vi "WPI_AccumulatorGetOutput.vi"(8 "error in (no error)":errorcluster, 11 "AIDeviceRef":T1={"DevStatus"={"status"=FALSE, "code"=0, "source"=""}, "Analog Channel"=enum."Invalid"}) -> (0 "error out":errorcluster, 1 "Duration (Seconds)":dbl, 2 "Value (Volt Seconds)":dbl, 3 "AIDeviceRef":T1={"DevStatus"={"status"=FALSE, "code"=0, "source"=""}, "Analog Channel"=enum."Invalid"})   [LabVIEW 2017]
doc: "Returns the current value of the accumulator on the FPGA on the robotRIO device. The GetOutput VI also returns the number of seconds that has passed since the accumulator was last reset. You can use this VI to perform averaging.\n\nThis software is licensed. Open the labview\\readme\\WPI Robotics Library Open Source License.txt file for more information."
uses:
  <vilib>/Rock Robotics/WPI/AnalogChannel/WPI_AnalogChannelDevRef.ctl
  <vilib>/Rock Robotics/SystemInterfaces/AI/FPGA_AIChannel.ctl
  <vilib>/Rock Robotics/SystemInterfaces/System/FPGA_SystemGet.vi
  <vilib>/Rock Robotics/SystemInterfaces/AI/FPGA_AIAverageBits.vi
  <vilib>/Rock Robotics/SystemInterfaces/AI/FPGA_AIERRInvalidAnalogChannel.vi
  <vilib>/Rock Robotics/SystemInterfaces/AI/FPGA_AIOversampleBits.vi
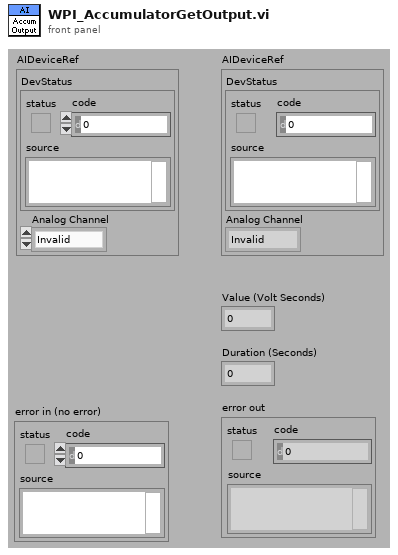
[diagram p1: front panel]
types:
  T1 = typedef "WPI_AnalogChannelDevRef.ctl" = cluster{"DevStatus":errorcluster, "Analog Channel":T2}
  T2 = typedef "FPGA_AIChannel.ctl" = enum8{"AI 0", "AI 1", "AI 2", "AI 3", "AI MXP 0", "AI MXP 1", "AI MXP 2", "AI MXP 3", "Invalid"}
  T3 = typedef "FPGA_AIDevRef.ctl" = cluster{"DevStatus":errorcluster}
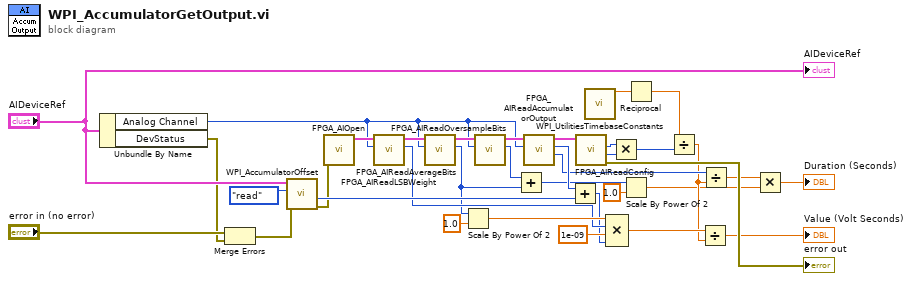
[diagram p0: block diagram]
diagram:
  n1 = Unbundle By Name("AIDeviceRef") -> ("Analog Channel"=w14:T2, "DevStatus"=w2:errorcluster)
  n2 = Merge Errors("error in (no error)", w2) -> (w1:errorcluster)
  n3 = call <vilib>:"WPI_AccumulatorOffset.vi"("error in (no error)"=w1, "Action"=enum16{"read", "write"}."read" ("what do"), "AIDeviceRef"="AIDeviceRef") -> ("error out"=w6:errorcluster, "Offset Out"=w31:i32)  [unwired: 1 in, 6 out]
  n4 = call <vilib>:"FPGA_AIOpen.vi"("error in (no error)"=w6) -> ("AI Reference out"=w28:T3)  [unwired: 2 in, 8 out]
  n5 = call <vilib>:"FPGA_AIReadLSBWeight.vi"("Channel"=w14, "AI Reference"=w28) -> ("LSBWeight"=w24:u32, "AI Reference"=w29:T3)  [unwired: 1 in, 7 out]
  n6 = call <vilib>:"FPGA_AIReadAverageBits.vi"("Channel"=w14, "AI Reference in"=w29) -> ("AverageBits"=w12:u8, "AI Reference out"=w16:T3)  [unwired: 1 in, 7 out]
  n7 = Scale By Power Of 2(n=w12, x=1.0) -> (x*2^n=w26:dbl)
  n8 = call <vilib>:"FPGA_AIReadOversampleBits.vi"("Channel"=w14, "AI Reference in"=w16) -> ("OversampleBits"=w13:u8, "AI Reference out"=w15:T3)  [unwired: 2 in, 6 out]
  n9 = Add(x=w13, y=w12) -> (x+y=w10:u8)
  n10 = call <vilib>:"FPGA_AIReadAccumulatorOutput.vi"("Channel"=w14, "AI Reference"=w15) -> ("Count"=w18:u32, "Value"=w32:i64, "AI Reference"=w22:T3)  [unwired: 1 in, 6 out]
  n11 = Add(x=w32, y=w31) -> (x+y=w23:i64)
  n12 = call <vilib>:"FPGA_AIReadConfig.vi"("AI Reference"=w22) -> ("error out"=→"error out":errorcluster, "Convert Rate"=w21:u32, "Scan Size"=w20:u8)  [unwired: 1 in, 7 out]
  n13 = call <vilib>:"WPI_UtilitiesTimebaseConstants.vi"() -> ("40 MHz FPGA clock"=w5:dbl)  [unwired: 13 in, 2 out]
  n14 = Compound Arithmetic op=MULTIPLY(w26, w24, 1e-09 ("y"), w23) -> (w19:dbl)
  n15 = Multiply(x=w20, y=w21) -> (x*y=w8:u32)
  n16 = Scale By Power Of 2(n=w10, x=1.0) -> (x*2^n=w9:dbl)
  n17 = Reciprocal(x=w5) -> (1/x=w4:dbl)
  n18 = Divide(x=w4, y=w8) -> (x/y=w17:dbl)
  n19 = Divide(x=w19, y=w17) -> (x/y=→"Value (Volt Seconds)":dbl)
  n20 = Divide(x=w18, y=w17) -> (x/y=w7:dbl)
  n21 = Multiply(x=w7, y=w9) -> (x*y=→"Duration (Seconds)":dbl)
  "AIDeviceRef" <- "AIDeviceRef"
